vi "DeInit.vi"(8 "error in (no error)":errorcluster, 11 "TranslationStageActor in":refnum<class "ArduinoTranslationStage.lvclass">) -> (0 "error out":errorcluster, 3 "TranslationStageActor out":refnum<class "ArduinoTranslationStage.lvclass">)   [LabVIEW 2023, in "ArduinoTranslationStage.lvlib" / "ArduinoTranslationStage.lvclass"]
uses:
  ArduinoTranslationStage.lvclass
  ArduinoTranslationStage.lvclass/ArduinoTranslationStage.ctl
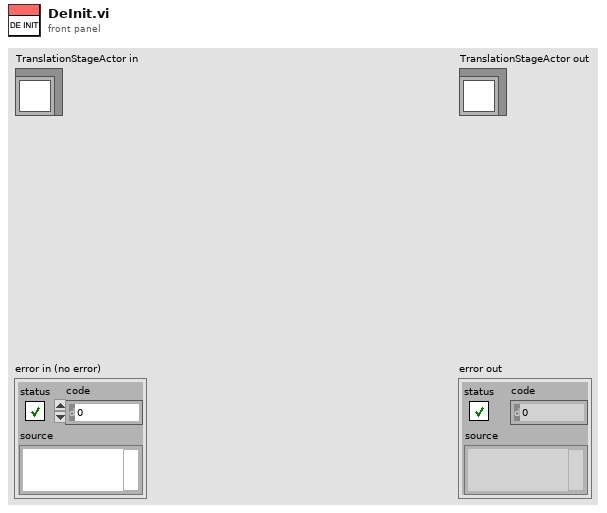
[diagram p1: front panel]
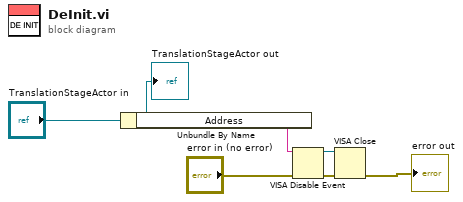
[diagram p0: block diagram]
diagram:
  n1 = Unbundle By Name("TranslationStageActor in") -> ("Address"=w1:string)
  n2 = VISA Disable Event(8:"error in (no error)", 11:w1) -> (0:w5:errorcluster, 3:w6:refnum<visa-resource-name>)  [unwired: 2 in]
  n3 = VISA Close(VISA resource name=w6, error in (no error)=w5) -> (error out=→"error out":errorcluster)
  "TranslationStageActor out" <- "TranslationStageActor in"
